vi "Start.vi"(8 "error in (no error)":errorcluster, 11 "PXImc Transceiver in":refnum<class "DSF PXImc Transceiver.lvclass">=refnum) -> (0 "error out":errorcluster, 3 "PXImc Transceiver out":refnum<class "DSF PXImc Transceiver.lvclass">)   [LabVIEW 2017, in "DSF Core.lvlib" / "DSF PXImc Transceiver.lvclass"]
uses:
  DSF PXImc Transceiver.lvclass
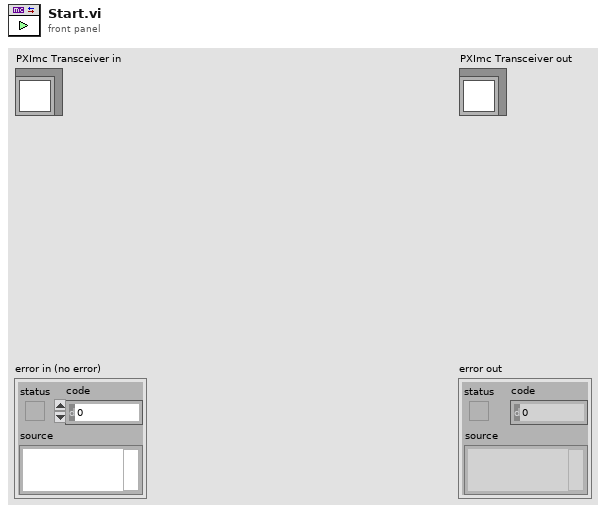
[diagram p1: front panel]
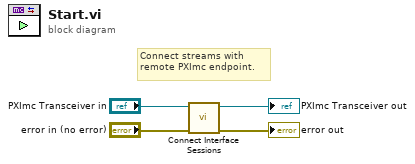
[diagram p0: block diagram]
diagram:
  # "Connect streams with remote PXImc endpoint."
  n1 = call "Connect Interface Sessions.vi"("error in (no error)"="error in (no error)", "PXImc Transceiver in"="PXImc Transceiver in") -> ("error out"=→"error out":errorcluster, "PXImc Transceiver out"=→"PXImc Transceiver out":refnum<class "DSF PXImc Transceiver.lvclass">)  [unwired: 8 in]
